vi "接收数据判断1.vi"(7 "上次正确接收数据时间":timestamp, 8 "错误输入（无错误）":errorcluster, 9 "IP地址比较位":bool, 10 "data out":string, 11 "队列输入":refnum<queue>) -> (0 "错误输出":errorcluster, 1 "结束标志位":bool, 2 "解析后数据":i32[][](array[numeric]), 3 "队列输出":refnum<queue>, 4 "正确接收数据时间":timestamp, 5 "状态显示":string)   [LabVIEW 2020]
panel:
  out "波形图表 6":i32[][](graph)
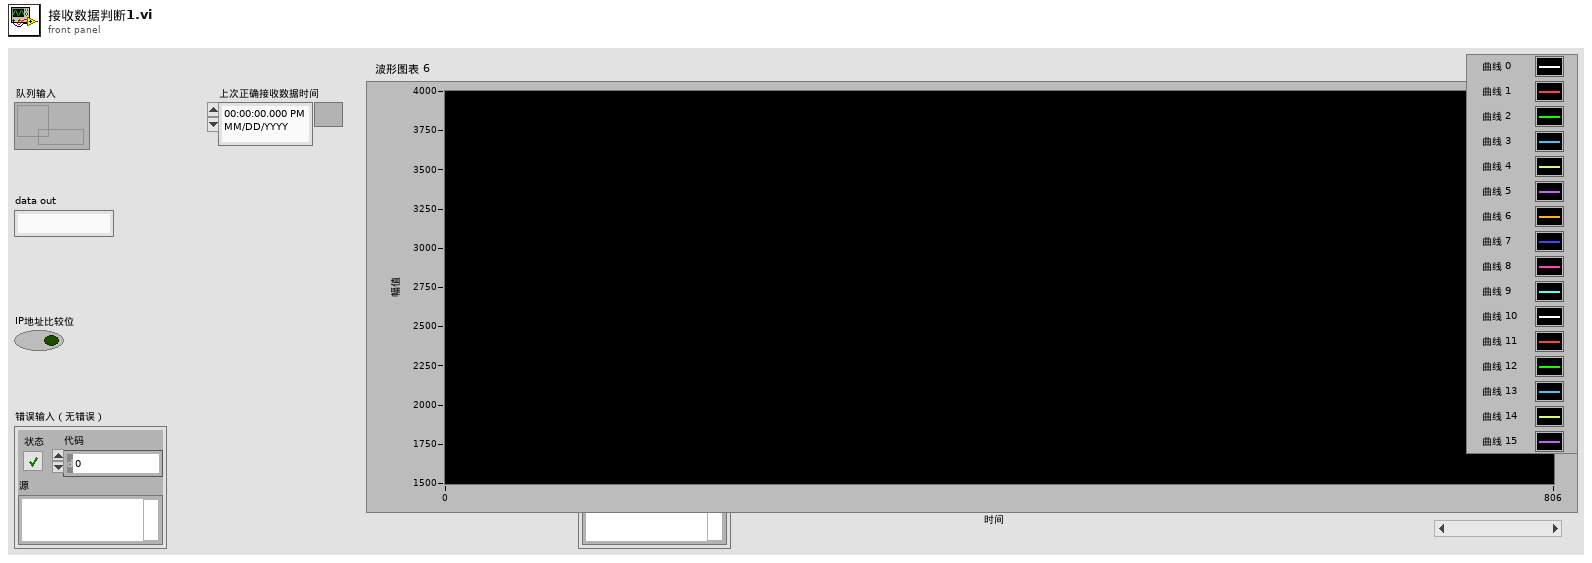
[diagram p1: front panel]
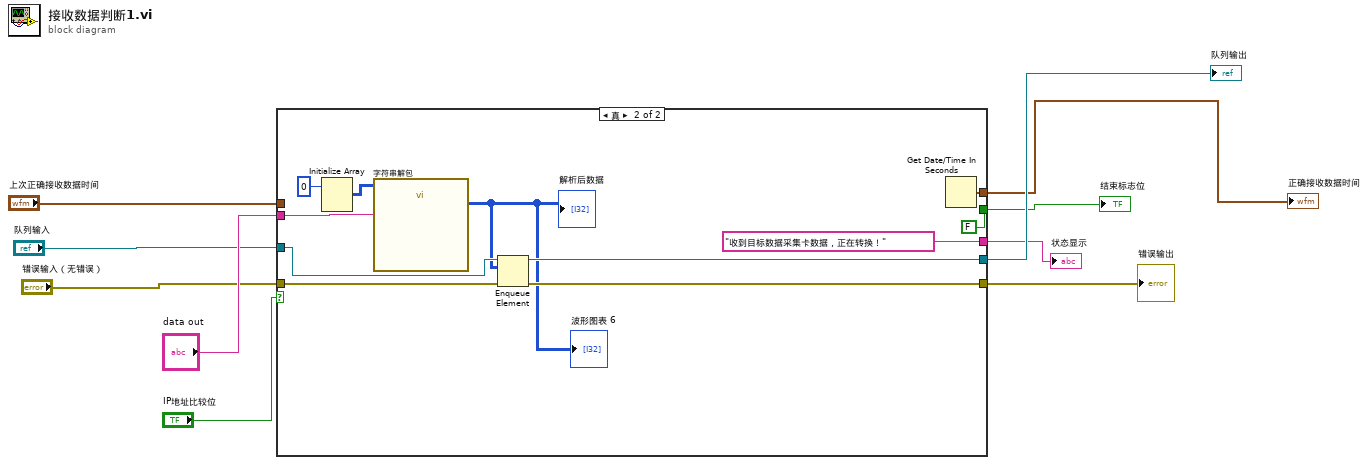
[diagram p0: block diagram]
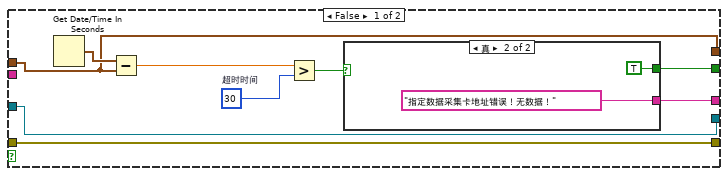
[diagram p2: hidden frame]
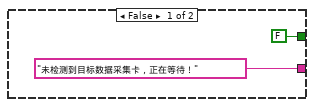
[diagram p3: hidden frame]
diagram:
  n1 = case shown="真" "IP地址比较位" {
    tunnel: "data out" -> [_ w32]
    tunnel: [w13 w31] -> w9
    tunnel: [w12 w30] -> w1
    tunnel: "队列输入" -> [w13 w29]
    tunnel: [w16 "收到目标数据采集卡数据，正在转换！"] -> w6
    tunnel: [w11 w27] -> w5
    tunnel: "上次正确接收数据时间" -> [w11 _]
    tunnel: [w14 FALSE] -> w3
    tunnel: "错误输入（无错误）" -> [w12 w26]
    frame False {
      w17 = u16 30  # 超时时间
      n2 = Get Date/Time In Seconds() -> (seconds since 1Jan1904=w19:timestamp)
      n3 = Subtract(x=w19, y=w11) -> (x-y=w18:dbl)
      n4 = Greater?(x=w18, y=w17) -> (0:w15:bool)
      n5 = case shown="真" w15 {
        tunnel: ["未检测到目标数据采集卡，正在等待！" "指定数据采集卡地址错误！无数据！"] -> w16
        tunnel: [FALSE TRUE] -> w14
        frame False {
        }
        frame True {
        }
      }
    }
    frame True {
      n6 = Initialize Array(0) -> (w33:i32[][])  [unwired: 2 in]
      n7 = call "字符串解包.vi"("输入数据"=w32, "初始化缓存"=w33) -> ("解析后数据"=w24:i32[][])  [unwired: 9 in]
      "解析后数据" <- w24
      "波形图表 6" <- w24
      n8 = Enqueue Element(queue=w29, element=w24, error in (no error)=w26) -> (queue out=w31:refnum<queue>, error out=w30:errorcluster)  [unwired: 1 in, 1 out]
      n9 = Get Date/Time In Seconds() -> (seconds since 1Jan1904=w27:timestamp)
    }
  }
  "错误输出" <- w1
  "结束标志位" <- w3
  "正确接收数据时间" <- w5
  "状态显示" <- w6
  "队列输出" <- w9
